vi "write_fifo.vi"(6 "buffers state in":T1=[{"depth"=0, "current read address"=0, "current write address"=0}, {"depth"=0, "current read address"=0, "current write address"=0}, {"depth"=0, "current read address"=0, "current write address"=0}], 7 "pixel-to-host\n mode":T3, 8 "FIFO overflow in":bool, 9 "maximum bit depth":i8, 10 "block index in":i32, 11 "values to be written":T4) -> (0 "FIFO overflow out":bool, 2 "block index out":i32, 3 "channels out":T4, 4 "buffers state out":T1)   [LabVIEW 2010]
uses:
  common_typedefs/channels_cluster.ctl
  common_typedefs/pixel_to_host_enum.ctl
  OnBoardBuffer/buffers_state_array.ctl
  OnBoardBuffer/buffer_state_cluster.ctl
  <vilib>/rvi/LocalResourceManager/LocalResourceManager.xnode
  <vilib>/rvi/DataTransferAndStorage/Container/Common/niFpgaContainerState.ctl
  <vilib>/rvi/DataTransferAndStorage/Container/Common/niFpgaDataTypeControl.ctl
  <vilib>/rvi/DataTransferAndStorage/Container/Common/niFpgaContainerImplementationControl.ctl
  <vilib>/rvi/DataTransferAndStorage/Container/Common/niFpgaContainerArbitrationOptionsControl.ctl
  <vilib>/rvi/DataTransferAndStorage/Container/Common/niFpgaTransferTypeControl.ctl
  <vilib>/rvi/DataTransferAndStorage/Container/Common/niFpgaContainerInitializationParameters.ctl
  <vilib>/rvi/Memory/Memory_Types/niFpgaMemoryInterfaceConfiguration.ctl
  <vilib>/rvi/FIFO/Fifo_Types/niFpgaFifoControlLogicControl.ctl
  <vilib>/rvi/DataTransferAndStorage/Container/Common/niFpgaContainerMetaDataKey.ctl
  <vilib>/rvi/DataTransferAndStorage/Container/XNode/niFpgaContainer.xnode
  <vilib>/rvi/DataTransferAndStorage/Container/Common/niFpgaContainerMethod.ctl
  <vilib>/rvi/DataTransferAndStorage/Container/Common/niFpgaContainerGetUniqueNameForEmu.vi
  <vilib>/rvi/DataTransferAndStorage/Container/Common/niFpgaContainerSetEmuInfo.vi
  <vilib>/rvi/eio/common/nirviEmuReportErrorAndStop.vi
  <vilib>/rvi/interface/RandomDataEmulation/nirviRandomDataFPGAFIFO.vi
  <vilib>/rvi/interface/RandomDataEmulation/niFpgaRandomDataHandleErrors.vi
  OnBoardBuffer/OnBoardBuffer.lvlib
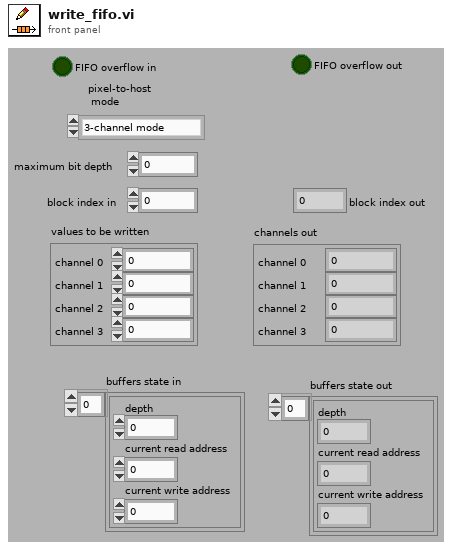
[diagram p1: front panel]
types:
  T1 = typedef "buffers_state_array.ctl" = T2[]
  T2 = typedef "OnBoardBuffer.lvlib/buffer_state_cluster.ctl" = cluster{"depth":u32, "current read address":u32, "current write address":u32}
  T3 = typedef "pixel_to_host_enum.ctl" = enum16{"3-channel mode", "4-channel mode"}
  T4 = typedef "channels_cluster.ctl" = cluster{"channel 0":u32, "channel 1":u32, "channel 2":u32, "channel 3":u32}
  T5 = typedef "niFpgaContainerMethod.ctl" = enum16{"<none>", "write", "read", "clear", "getNumberOfElementsToWrite", "getNumberOfElementsToRead", "enable", "disable", "flushAndDisable", "getStreamState", "readA", "readB", "dramWrite", "dramWriteWithByteEnables", "dramRequestData", "dramRetrieveData"}
  T6 = typedef "niFpgaTransferTypeControl.ctl" = enum16{"Target-Scoped", "Host to Target - DMA", "Target to Host - DMA", "Peer to Peer Reader", "Peer to Peer Writer", "Bidirectional"}
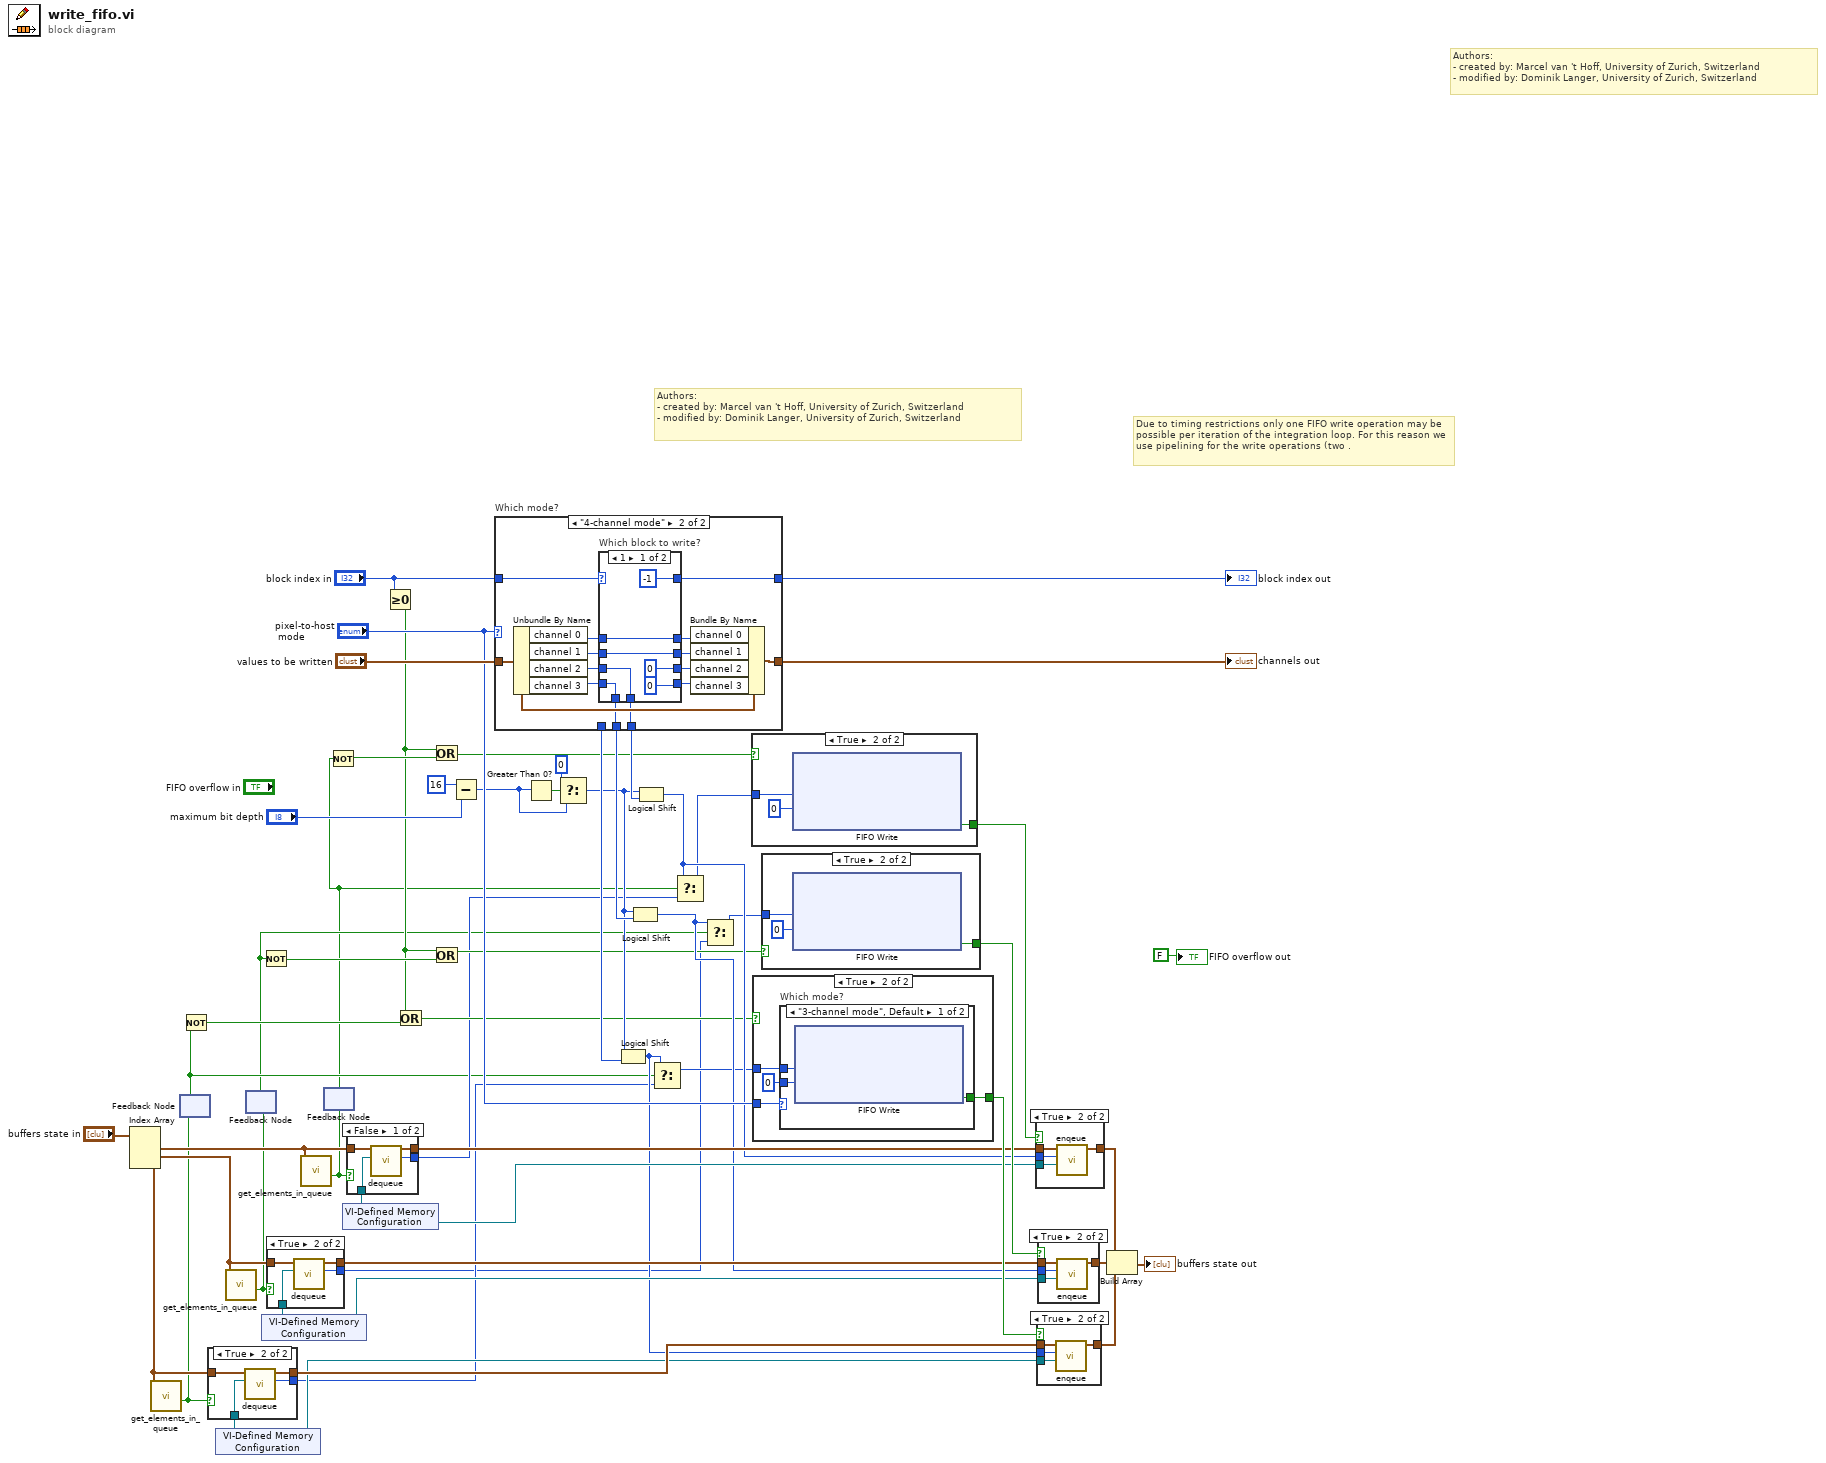
[diagram p0: block diagram]
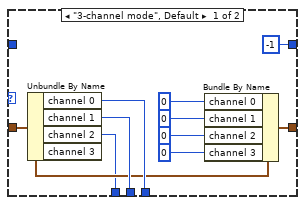
[diagram p12: hidden frame]
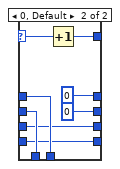
[diagram p13: hidden frame]
diagram:
  # "Due to timing restrictions only one FIFO write operation may be possible per iteration of the integration loop. For this reason we use pipelining for the write operations (two ."
  # "Authors: \n- created by: Marcel van 't Hoff, University of Zurich, Switzerland\n- modified by: Dominik Langer, University of Zurich, Switzerland"
  # "Authors: \n- created by: Marcel van 't Hoff, University of Zurich, Switzerland\n- modified by: Dominik Langer, University of Zurich, Switzerland"
  n1 = Index Array(array="buffers state in") -> (element #1=w31:T2, element #2=w29:T2, element #3=w27:T2)  [unwired: 3 in]
  n2 = call "get_elements_in_queue.vi"("on-board buffer in"=w27) -> ("empty?"=w8:bool)  [unwired: 9 in, 1 out]
  n3 = feedback-in #1(w8) -> ()
  n4 = feedback #1() -> (w3:bool)  [unwired: 1 in]
  n5 = Not(x=w3) -> (.not. x?=w12:bool)
  n6 = xnode "VI-Defined Memory Configuration"() -> ("Memory Out"=w24:refnum<k21>)
  n7 = case shown="True" w8 {
    tunnel: w27 -> [w55 w59]
    tunnel: [w55 w58] -> w26
    tunnel: w24 -> [_ w57]
    tunnel: [_ w56] -> w5
    frame False {
    }
    frame True {
      n8 = call "dequeue.vi"("memory ref"=w57, "on-board buffer in"=w59) -> ("data"=w56:u16, "on-board buffer out"=w58:T2)  [unwired: 8 in]
    }
  }
  n9 = call "get_elements_in_queue.vi"("on-board buffer in"=w29) -> ("empty?"=w9:bool)  [unwired: 9 in, 1 out]
  n10 = feedback-in #2(w9) -> ()
  n11 = feedback #2() -> (w2:bool)  [unwired: 1 in]
  n12 = Not(x=w2) -> (.not. x?=w13:bool)
  n13 = xnode "VI-Defined Memory Configuration"() -> ("Memory Out"=w23:refnum<k21>)
  n14 = case shown="True" w9 {
    tunnel: w29 -> [w60 w64]
    tunnel: [w60 w63] -> w28
    tunnel: w23 -> [_ w62]
    tunnel: [_ w61] -> w4
    frame False {
    }
    frame True {
      n15 = call "dequeue.vi"("memory ref"=w62, "on-board buffer in"=w64) -> ("data"=w61:u16, "on-board buffer out"=w63:T2)  [unwired: 8 in]
    }
  }
  n16 = call "get_elements_in_queue.vi"("on-board buffer in"=w31) -> ("empty?"=w7:bool)  [unwired: 9 in, 1 out]
  n17 = feedback-in #3(w7) -> ()
  n18 = feedback #3() -> (w1:bool)  [unwired: 1 in]
  n19 = Not(x=w1) -> (.not. x?=w16:bool)
  n20 = xnode "VI-Defined Memory Configuration"() -> ("Memory Out"=w25:refnum<k21>)
  n21 = case shown="False" w7 {
    tunnel: w31 -> [w68 w69]
    tunnel: [w67 w69] -> w30
    tunnel: w25 -> [w66 _]
    tunnel: [w65 _] -> w6
    frame False {
      n22 = call "dequeue.vi"("memory ref"=w66, "on-board buffer in"=w68) -> ("data"=w65:u16, "on-board buffer out"=w67:T2)  [unwired: 8 in]
    }
    frame True {
    }
  }
  n23 = Greater Or Equal To 0?(x="block index in") -> (x >= 0?=w11:bool)
  n24 = Or(x=w11, y=w12) -> (x .or. y?=w10:bool)
  n25 = Or(x=w11, y=w16) -> (x .or. y?=w15:bool)
  n26 = Or(x=w11, y=w13) -> (x .or. y?=w14:bool)
  n27 = Subtract(x=i8 16, y="maximum bit depth") -> (x-y=w43:i8)
  n28 = case "Which mode?" shown="\"4-channel mode\"" "pixel-to-host\n mode" {
    tunnel: [w73 w83] -> w50
    tunnel: "block index in" -> [_ w80]
    tunnel: "values to be written" -> [w72 w85]
    tunnel: [-1 ("block index in") w84] -> w54
    tunnel: [w78 w82] -> w41
    tunnel: [w79 w81] -> w40
    tunnel: [w70 _] -> w39
    frame "3-channel mode", Default {
      n29 = Unbundle By Name(w72) -> ("channel 0"=w79:u32, "channel 1"=w78:u32, "channel 2"=w70:u32)  [unwired: 1 out]
      n30 = Bundle By Name(cluster=w72, "channel 0"=u32 0, "channel 1"=u32 0, "channel 2"=u32 0 ("channel 0"), "channel 3"=u32 0 ("channel 1")) -> (w73:T4)
    }
    frame "4-channel mode" {
      n31 = Unbundle By Name(w85) -> ("channel 0"=w86:u32, "channel 1"=w87:u32, "channel 2"=w88:u32, "channel 3"=w89:u32)
      n32 = case "Which block to write?" shown="1" w80 {
        selector: w80 -> [_ w101]
        tunnel: [w100 w108] -> w81
        tunnel: w86 -> [w98 w108]
        tunnel: [w99 w107] -> w82
        tunnel: w87 -> [w97 w107]
        tunnel: w88 -> [w100 w106]
        tunnel: w89 -> [w99 w105]
        tunnel: [u32 0 ("channel 2") w106] -> w91
        tunnel: [u32 0 ("channel 3") w105] -> w90
        tunnel: [w98 u32 0 ("channel 0")] -> w92
        tunnel: [w97 u32 0 ("channel 1")] -> w93
        tunnel: [-1 ("block index in") w102] -> w84
        frame 1 {
        }
        frame 0, Default {
          n33 = Increment(x=w101) -> (x+1=w102:i32)
        }
      }
      n34 = Bundle By Name(cluster=w85, "channel 0"=w92, "channel 1"=w93, "channel 2"=w91, "channel 3"=w90) -> (w83:T4)
    }
  }
  "channels out" <- w50
  "block index out" <- w54
  n35 = Greater Than 0?(x=w43) -> (x > 0?=w42:bool)
  n36 = Select(t=i8 0 ("f"), s=w42, f=w43) -> (s? t:f=w38:i8)
  n37 = Logical Shift(y=w38, x=w39) -> (x << y=w18:u32)
  n38 = Logical Shift(y=w38, x=w41) -> (x << y=w19:u32)
  n39 = Logical Shift(y=w38, x=w40) -> (x << y=w22:u32)
  n40 = Select(t=w18, s=w3, f=w5) -> (s? t:f=w17:u32)
  n41 = Select(t=w22, s=w1, f=w6) -> (s? t:f=w21:u32)
  n42 = Select(t=w19, s=w2, f=w4) -> (s? t:f=w20:u32)
  n43 = case shown="True" w15 {
    tunnel: w21 -> [_ w110]
    tunnel: [_ w109] -> w37
    frame False {
    }
    frame True {
      n44 = xnode ("FIFO Write")("Element"=w110, "Timeout"=0) -> ("Timed Out?"=w109:bool)  [unwired: 1 in, 1 out]
    }
  }
  n45 = case shown="True" w10 {
    tunnel: "pixel-to-host\n mode" -> [_ w143]
    tunnel: [_ w142] -> w35
    tunnel: w17 -> [_ w141]
    frame False {
    }
    frame True {
      n46 = case "Which mode?" shown="\"3-channel mode\", Default" w143 {
        tunnel: [w146 _] -> w142
        tunnel: w141 -> [w145 _]
        tunnel: 0 ("Timeout") -> [w144 _]
        frame "3-channel mode", Default {
          n47 = xnode ("FIFO Write")("Element"=w145, "Timeout"=w144) -> ("Timed Out?"=w146:bool)  [unwired: 1 in, 1 out]
        }
        frame "4-channel mode" {
        }
      }
    }
  }
  n48 = case shown="True" w14 {
    tunnel: [_ w177] -> w36
    tunnel: w20 -> [_ w176]
    frame False {
    }
    frame True {
      n49 = xnode ("FIFO Write")("Element"=w176, "Timeout"=0) -> ("Timed Out?"=w177:bool)  [unwired: 1 in, 1 out]
    }
  }
  n50 = case shown="True" w37 {
    tunnel: w30 -> [w206 w210]
    tunnel: w22 -> [_ w209]
    tunnel: [w206 w208] -> w34
    tunnel: w25 -> [_ w207]
    frame False {
    }
    frame True {
      n51 = call "enqeue.vi"("memory ref"=w207, "data"=w209, "buffer state in"=w210) -> ("buffer state out"=w208:T2)  [unwired: 8 in]
    }
  }
  n52 = case shown="True" w35 {
    tunnel: w18 -> [_ w215]
    tunnel: w26 -> [w211 w214]
    tunnel: [w211 w213] -> w33
    tunnel: w24 -> [_ w212]
    frame False {
    }
    frame True {
      n53 = call "enqeue.vi"("memory ref"=w212, "data"=w215, "buffer state in"=w214) -> ("buffer state out"=w213:T2)  [unwired: 8 in]
    }
  }
  n54 = case shown="True" w36 {
    tunnel: w19 -> [_ w220]
    tunnel: w28 -> [w216 w219]
    tunnel: [w216 w218] -> w32
    tunnel: w23 -> [_ w217]
    frame False {
    }
    frame True {
      n55 = call "enqeue.vi"("memory ref"=w217, "data"=w220, "buffer state in"=w219) -> ("buffer state out"=w218:T2)  [unwired: 8 in]
    }
  }
  n56 = Build Array(w34, w32, w33) -> (→"buffers state out":T2[])
  "FIFO overflow out" <- FALSE ("FIFO overflow in")
